vi "1. Color Class and Pattern Match_WorkOrderBoard.vi"() -> ()   [LabVIEW 2019]
doc: "c 2020 ReMiSYS All rights reserved."
panel:
  out "cutImage":T1(plugin-control)
  out "ArrayOut":u32[][](array[colorbox])
  out "appended path":path
  out "Input Image":T1(plugin-control)
  in  "Stop (F)":bool caption="Stop"
  in  "Loop Delay (ms)":u32(slide)=1000 scale=0.0..1500.0
  # "c 2022 ReMiSYS All rights reserved."
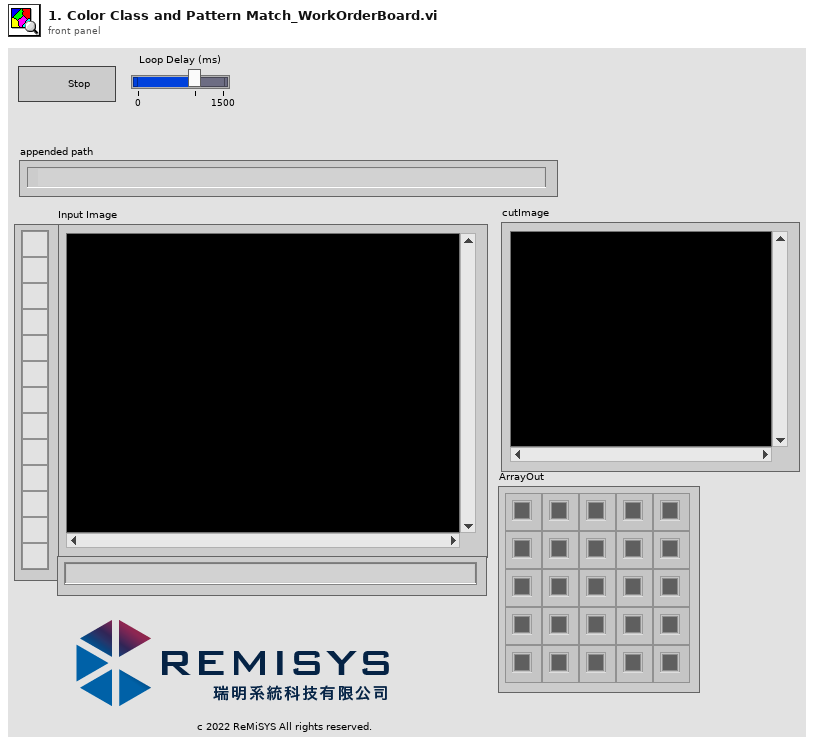
[diagram p1: front panel]
types:
  T1 = typedef "IMAQ Image.ctl" = refnum<image>
  T2 = cluster{"Global Rectangle":i32[], "Contours":cluster{"ID":enum32{"External", "Internal"}, "Type":u32, "Coordinates":i32[]}[]}
  T3 = cluster{"ID":enum32{"External", "Internal"}, "Type":u32, "Coordinates":i32[]}
  T4 = typedef "IMAQ GM Match Report.ctl" = cluster{"Position":cluster{"x":sgl, "y":sgl}, "Angle":sgl, "Scale":sgl, "Score":sgl, "Bounding Box":cluster{"x":sgl, "y":sgl}[], "Contrast Reversed":bool, "Occlusion %":sgl, "Template Target Curve Score":sgl, "Target Template Curve Score":sgl, "Correlation Score":sgl}
  T5 = cluster{"ID":enum32{"External", "Internal"}, "Type":u32, "Coordinates":i32[]}[]
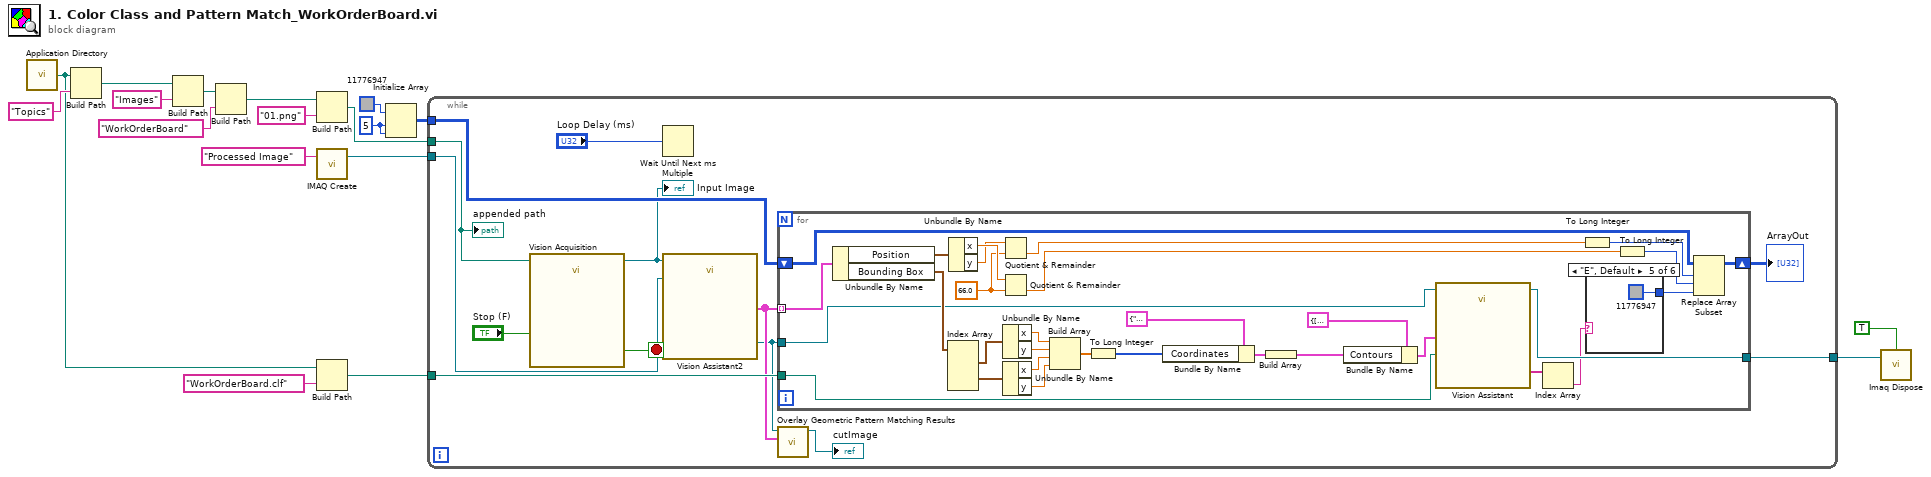
[diagram p0: block diagram]
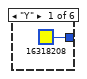
[diagram p2: hidden frame]
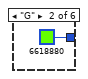
[diagram p3: hidden frame]
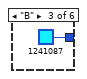
[diagram p4: hidden frame]
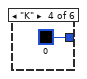
[diagram p5: hidden frame]
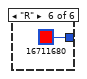
[diagram p6: hidden frame]
diagram:
  w2 = 5 ("dimension size")
  n1 = call <vilib>:"Application Directory.vi"() -> ("Application Directory"=w4:path)
  n2 = Build Path(base path=w4, name or relative path="Topics") -> (appended path=w15:path)
  n3 = Build Path(base path=w15, name or relative path="Images") -> (appended path=w7:path)
  n4 = Build Path(base path=w7, name or relative path="WorkOrderBoard") -> (appended path=w8:path)
  n5 = Build Path(base path=w8, name or relative path="01.png") -> (appended path=w12:path)
  n6 = call "IMAQ Create"("Image Name"="Processed Image") -> ("New Image"=w18:T1)  [unwired: 3 in, 2 out]
  n7 = Build Path(base path=w4, name or relative path="WorkOrderBoard.clf") -> (appended path=w5:path)
  n8 = Initialize Array(u32 11776947 ("Color Box"), w2, w2) -> (w1:u32[][])
  n9 = while {
    tunnel: w18 -> [w27]
    tunnel: w12 -> [w28]
    tunnel: [w24] -> w11
    tunnel: w5 -> [w25]
    tunnel: w1 -> [w26]
    stop <- w31 stop-if-true
    n10 = call "Vision Acquisition"("Image Path"=w28, "Stop (F)"="Stop (F)") -> ("Image Out"=w21:T1, "Stopped"=w31:bool)  [unwired: 1 in, 23 out]
    "Input Image" <- w21
    n11 = Wait Until Next ms Multiple(millisecond multiple="Loop Delay (ms)") -> ()  [unwired: 1 out]
    n12 = call "Vision Assistant2"("Image In"=w21, "Image Dst"=w27) -> ("Matches (Pattern Matching 1)"=w22:T4[], "Image Buffer (Image Buffer 2)"=w20:T1)  [unwired: 21 in, 3 out]
    n13 = for {
      tunnel: w22 -> [w62] mode=indexing
      tunnel: w25 -> [w57]
      tunnel: [w56] -> w24
      tunnel: w20 -> [w37]
      shift-right: [w38] -> w23
      shift-left: w26 -> [w55]
      w59 = sgl 66.0 ("y")
      n14 = Unbundle By Name(w62) -> ("Position"=w61:cluster{"x":sgl, "y":sgl}, "Bounding Box"=w54:cluster{"x":sgl, "y":sgl}[])
      n15 = Index Array(array=w54) -> (element #1=w53:cluster{"x":sgl, "y":sgl}, element #3=w52:cluster{"x":sgl, "y":sgl})  [unwired: 4 in, 2 out]
      n16 = Unbundle By Name(w61) -> ("x"=w60:sgl, "y"=w58:sgl)
      n17 = Quotient & Remainder(x=w58, y=w59) -> (floor(x/y)=w34:sgl)  [unwired: 1 out]
      n18 = Quotient & Remainder(x=w60, y=w59) -> (floor(x/y)=w36:sgl)  [unwired: 1 out]
      n19 = Unbundle By Name(w53) -> ("x"=w49:sgl, "y"=w48:sgl)
      n20 = Unbundle By Name(w52) -> ("x"=w47:sgl, "y"=w46:sgl)
      n21 = Build Array(w49, w48, w47, w46) -> (w45:sgl[])
      n22 = To Long Integer(number=w45) -> (32bit integer=w44:i32[])
      n23 = Bundle By Name(cluster=T3 {"ID"=enum."External", "Type"=3, "Coordinates"=[]}, "Coordinates"=w44) -> (w43:T3)
      n24 = Build Array(w43) -> (w42:T5)
      n25 = Bundle By Name(cluster=T2 {"Global Rectangle"=[204, 68, 525, 390], "Contours"=[]} ("ROI Descriptor (Color Classification 1)"), "Contours"=w42) -> (w51:T2)
      n26 = call "Vision Assistant"("Image In"=w37, "ROI Descriptor (Color Classification 1)"=w51, "File Path (Color Classification 1)"=w57) -> ("Image Out"=w56:T1, "Classes (Color Classification 1)"=w41:string[])  [unwired: 22 in, 1 out]
      n27 = Index Array(array=w41) -> (element=w40:string)  [unwired: 1 in]
      n28 = To Long Integer(number=w34) -> (32bit integer=w33:i32)
      n29 = case shown="\"E\", Default" w40 {
        tunnel: [u32 16318208 ("Color Box") u32 6618880 ("Color Box") u32 1241087 ("Color Box") u32 0 ("Color Box") u32 11776947 ("Color Box") u32 16711680 ("Color Box")] -> w39
        frame "Y" {
        }
        frame "G" {
        }
        frame "B" {
        }
        frame "K" {
        }
        frame "E", Default {
        }
        frame "R" {
        }
      }
      n30 = To Long Integer(number=w36) -> (32bit integer=w35:i32)
      n31 = Replace Array Subset(array=w55, new element=w39, index (row)=w33, index (col)=w35) -> (w38:u32[][])
    }
    "ArrayOut" <- w23
    n32 = call "Overlay Geometric Pattern Matching Results.vi"("Matches"=w22, "Image"=w20) -> ("Image Out"=→"cutImage":T1)  [unwired: 8 in, 1 out]
    "appended path" <- w28
  }
  n33 = call "Imaq Dispose"("All Images? (No)"=TRUE, "Image"=w11) -> ()  [unwired: 4 in, 1 out]
